vi "OSTest.vi"() -> ()   [LabVIEW 2012]
uses:
  <instrlib>/Ocean Server OS4000/Ocean Server OS4000.lvlib
panel:
  out "VISA resource name out":refnum<visa-resource-name>
  out "error out":errorcluster
  in  "VISA resource name":refnum<visa-resource-name>
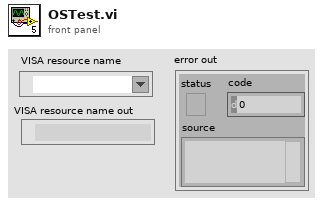
[diagram p1: front panel]
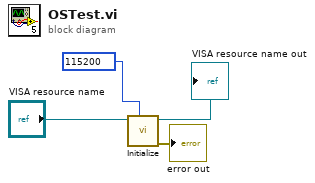
[diagram p0: block diagram]
diagram:
  w4 = u32 115200 items=["4800", "9600", "14400", "19200", "38400", "57600", "115200"]
  n1 = call <instrlib>:"Initialize.vi"("Baud Rate"=w4, "VISA resource name"="VISA resource name") -> ("error out"=→"error out":errorcluster, "VISA resource name out"=→"VISA resource name out":refnum<visa-resource-name>)  [unwired: 8 in]
